vi "MyrioProject.vi"() -> ()   [LabVIEW 2018]
doc: "The myRIO Project template acquires acceleration data from the onboard accelerometer and displays the changes of acceleration values in a waveform chart."
uses:
  <vilib>/myRIO/Common/Instrument Driver Framework/myRIO v1.0/Encoder/typedefs/Encoder Signal Mode.ctl
  <vilib>/Platform/TimedLoop/XDataNode/timing_clust.ctl
  <vilib>/Platform/TimedLoop/XDataNode/nitl_modes.ctl
  <vilib>/Platform/TimedLoop/XDataNode/wakeup.ctl
  <vilib>/Analysis/Matrix/Datatypes/RealMatrix.ctl
  <vilib>/myRIO/Instrument Drivers/Onboard IO/PWM/typedefs/PWM Reference.ctl
  <vilib>/myRIO/Common/Instrument Driver Framework/Utilities/typedefs/myRIO Generic Hardware Reference.ctl
  <vilib>/myRIO/Common/Instrument Driver Framework/Utilities/typedefs/Hardware Version Enum.ctl
  <vilib>/myRIO/Common/Instrument Driver Framework/Utilities/typedefs/myRIO v1.0 Reference.ctl
  <vilib>/myRIO/Common/Instrument Driver Framework/Utilities/typedefs/Generic FPGA Reference.ctl
  <vilib>/myRIO/Common/Instrument Driver Framework/myRIO v1.0/PWM/typedefs/PWM Channels Enum.ctl
  <vilib>/myRIO/Instrument Drivers/Onboard IO/PWM/typedefs/PWM Configuration.ctl
  <vilib>/userdefined/High Color/nirio_resource_hc.ctl
  <vilib>/myRIO/Common/Instrument Driver Framework/myRIO v1.0/Encoder/typedefs/Encoder Configuration v1.0.ctl
  <vilib>/myRIO/Instrument Drivers/Onboard IO/Encoder/typedefs/Encoder Reference.ctl
  <vilib>/myRIO/Common/Instrument Driver Framework/myRIO v1.0/Encoder/typedefs/Encoder Channels Enum.ctl
  <vilib>/myRIO/Instrument Drivers/Onboard IO/DIO/typedefs/DIO Reference.ctl
  <vilib>/myRIO/Common/Instrument Driver Framework/myRIO v1.0/DIO/typedefs/DIO Channels List.ctl
  <vilib>/myRIO/Common/Instrument Driver Framework/myRIO v1.0/DIO/typedefs/DIO Channels Enum.ctl
  <vilib>/myRIO/Instrument Drivers/Onboard IO/AI/typedefs/AI Reference.ctl
  <vilib>/myRIO/Common/Instrument Driver Framework/myRIO v1.0/AI/typedefs/AI Channels List.ctl
  <vilib>/myRIO/Common/Instrument Driver Framework/myRIO v1.0/AI/typedefs/AI Channels Enum.ctl
  <vilib>/myRIO/Common/Instrument Driver Framework/Utilities/typedefs/Analog Scaling Constants List.ctl
  <vilib>/myRIO/Common/Instrument Driver Framework/Utilities/typedefs/Analog Scaling Constants.ctl
  <vilib>/myRIO/Common/Instrument Driver Framework/myRIO v1.0/PWM/vis/myRIO v1.1 Open PWM.vi
  <vilib>/myRIO/Common/Instrument Driver Framework/myRIO v1.0/Encoder/vis/myRIO v1.1 Open Encoder.vi
  <vilib>/myRIO/Common/Instrument Driver Framework/Utilities/vis/Is FPGA Ref Available.vi
  <vilib>/myRIO/Common/Instrument Driver Framework/myRIO v1.0/AI/vis/myRIO v1.1 Open AI.vi
  <vilib>/myRIO/Common/Instrument Driver Framework/myRIO v1.0/DIO/vis/myRIO v1.1 Open DIO.vi
  <vilib>/myRIO/Instrument Drivers/Onboard IO/PWM/vis/Set Duty Cycle and Frequency.vi
  <vilib>/myRIO/Instrument Drivers/Onboard IO/DIO/vis/Write.vi
  <vilib>/myRIO/Common/Instrument Driver Framework/Utilities/vis/Validate Channels.vi
  <vilib>/myRIO/Common/Instrument Driver Framework/myRIO v1.0/PWM/vis/myRIO v1.0 Reserve PWM.vi
  <vilib>/myRIO/Common/Instrument Driver Framework/myRIO v1.0/Encoder/vis/myRIO v1.0 Reserve Encoder.vi
  <vilib>/myRIO/Common/Instrument Driver Framework/myRIO v1.0/AI/vis/myRIO v1.0 Reserve AI.vi
  <vilib>/myRIO/Common/Instrument Driver Framework/myRIO v1.0/DIO/vis/myRIO v1.0 Reserve DIO.vi
  <vilib>/myRIO/Common/Instrument Driver Framework/myRIO v1.0/Encoder/vis/myRIO v1.0 Close Encoder.vi
  <vilib>/myRIO/Common/Instrument Driver Framework/myRIO v1.0/PWM/vis/myRIO v1.0 Close PWM.vi
  <vilib>/myRIO/Common/Instrument Driver Framework/myRIO v1.0/PWM/vis/myRIO v1.0 Build MUX Configuration PWM.vi
  <vilib>/myRIO/Common/Instrument Driver Framework/myRIO v1.0/Resource Manager/vis/myRIO v1.0 Reserve Channel List.vi
  <vilib>/myRIO/Common/Instrument Driver Framework/myRIO v1.0/Encoder/vis/myRIO v1.0 Build MUX Configuration Encoder.vi
  <vilib>/myRIO/Common/Instrument Driver Framework/myRIO v1.0/AI/vis/myRIO v1.0 Build MUX Configuration AI.vi
  <vilib>/myRIO/Common/Instrument Driver Framework/myRIO v1.0/DIO/vis/myRIO v1.0 Build MUX Configuration DIO.vi
  <vilib>/myRIO/Common/Instrument Driver Framework/myRIO v1.0/Encoder/vis/myRIO v1.0 Unreserve Encoder.vi
  <vilib>/myRIO/Common/Instrument Driver Framework/myRIO v1.0/PWM/vis/myRIO v1.0 Unreserve PWM.vi
  <vilib>/myRIO/Common/Instrument Driver Framework/myRIO v1.0/Resource Manager/vis/myRIO v1.0 Create Configuration List.vi
  <vilib>/myRIO/Common/Instrument Driver Framework/myRIO v1.0/Resource Manager/vis/myRIO v1.0 Reserve Channel.vi
  <vilib>/myRIO/Common/Instrument Driver Framework/myRIO v1.0/Resource Manager/vis/myRIO v1.0 Unreserve Channel.vi
  <vilib>/myRIO/Common/Instrument Driver Framework/myRIO v1.0/Resource Manager/vis/myRIO v1.0 Unreserve Channel List.vi
  <vilib>/myRIO/Common/Instrument Driver Framework/myRIO v1.0/Resource Manager/vis/myRIO v1.0 Build Mutex Name.vi
  <vilib>/Utility/VariantDataType/GetNumericInfo.vi
  <vilib>/Utility/error.llb/Error Cluster From Error Code.vi
  <vilib>/myRIO/Common/Instrument Driver Framework/myRIO v1.0/myRIO v1.1 Open.vi
  <vilib>/myRIO/Common/Instrument Driver Framework/Utilities/vis/IO Manager.vi
  <vilib>/myRIO/Common/Instrument Driver Framework/Utilities/vis/Configuration Manager.vi
  <vilib>/myRIO/Common/Instrument Driver Framework/myRIO v1.0/Resource Manager/vis/myRIO v1.0 Configure IO.vi
  <vilib>/myRIO/Common/Instrument Driver Framework/myRIO v1.0/myRIO v1.0 Close.vi
  <vilib>/myRIO/Common/Instrument Driver Framework/myRIO v1.0/PWM/vis/myRIO v1.0 Write PWM.vi
  <vilib>/myRIO/Common/Instrument Driver Framework/myRIO v1.0/Encoder/vis/myRIO v1.0 Configure Encoder.vi
  <vilib>/myRIO/Common/Instrument Driver Framework/myRIO v1.0/Encoder/vis/myRIO v1.0 Enable Encoder.vi
  <vilib>/myRIO/Common/Instrument Driver Framework/myRIO v1.0/DIO/vis/myRIO v1.0 Read DIO.vi
  <vilib>/myRIO/Common/Instrument Driver Framework/myRIO v1.0/AI/vis/myRIO v1.0 Get Scaling Constants AI.vi
  <vilib>/myRIO/Common/Instrument Driver Framework/myRIO v1.0/AI/vis/myRIO v1.0 Read AI.vi
  <vilib>/myRIO/Common/Instrument Driver Framework/myRIO v1.0/Encoder/vis/myRIO v1.0 Read Encoder.vi
  <vilib>/myRIO/Common/Instrument Driver Framework/myRIO v1.0/DIO/vis/myRIO v1.0 Write DIO.vi
  <vilib>/myRIO/Common/Instrument Driver Framework/myRIO v1.0/Encoder/vis/myRIO v1.0 Shutdown Encoder.vi
  <vilib>/myRIO/Common/Instrument Driver Framework/myRIO v1.0/PWM/vis/myRIO v1.0 Shutdown PWM.vi
  <vilib>/platform/TimedLoop/XDataNode/XDataNode.xnode
  <vilib>/myRIO/Instrument Drivers/Onboard IO/PWM/vis/myRIO PWM Open.xnode
  <vilib>/myRIO/Instrument Drivers/Onboard IO/Encoder/vis/myRIO Encoder Open.xnode
  <vilib>/myRIO/Express VI/Onboard Devices/Button/Button Express VI.xnode
  <vilib>/myRIO/Instrument Drivers/Onboard IO/DIO/vis/myRIO DIO Open.xnode
  <vilib>/myRIO/Express VI/Onboard IO/AI/AI Express VI.xnode
  <vilib>/myRIO/Instrument Drivers/Onboard IO/AI/vis/myRIO AI Open.xnode
  <vilib>/myRIO/Express VI/Onboard IO/PWM/PWM Express VI.xnode
  <vilib>/myRIO/Express VI/Onboard IO/DO/DO Express VI.xnode
  <vilib>/myRIO/Instrument Drivers/Onboard IO/Encoder/Encoder.lvlib
  <vilib>/myRIO/Instrument Drivers/Onboard IO/PWM/PWM.lvlib
  <vilib>/myRIO/Instrument Drivers/Onboard IO/DIO/DIO.lvlib
  <vilib>/myRIO/Instrument Drivers/Onboard IO/AI/AI.lvlib
  <vilib>/Platform/TimedLoop/XDataNode/XDNodeRunTimeDep.lvlib
  <vilib>/Analysis/Matrix/NI_Matrix.lvlib
panel:
  out "Waveform Chart 2":cluster{"velocidad":dbl, "Numeric out":dbl}(graph)
  out "Waveform Chart":cluster{"velocidad":dbl, "Numeric out":dbl}(graph)
  in  "pequeoffset":dbl
  in  "s":bool
  in  "grandeoffset":dbl
  in  "saturacion 2":dbl=0.3
  in  "Garra":bool
  out "stall":bool
  in  "Start":bool
  in  "Stop Button":bool
  out "element":dbl
  out "element 2":dbl
  in  "manual":bool
  out "data":dbl
  out "sensor2 (A/AI2 (Pin 7))":dbl
  out "sensor1":dbl
  out "stallRojo (A/AI0 (Pin 3))":dbl
  out "stallBlanco (A/AI1 (Pin 5))":dbl
  out "subarray 2":dbl[][](array[numeric])
  out "subarray":dbl[][](array[numeric])
  out "vectores":dbl[][][](array[numeric])
  in  "saturacion":dbl=0.3
  in  "Garra":dbl(slide)=0.5 scale=0.05..0.1
  in  "Subir":dbl(slide)=0.5 scale=0.05..0.15
  in  "Reset Counter 2":bool
  in  "Reset Counter":bool
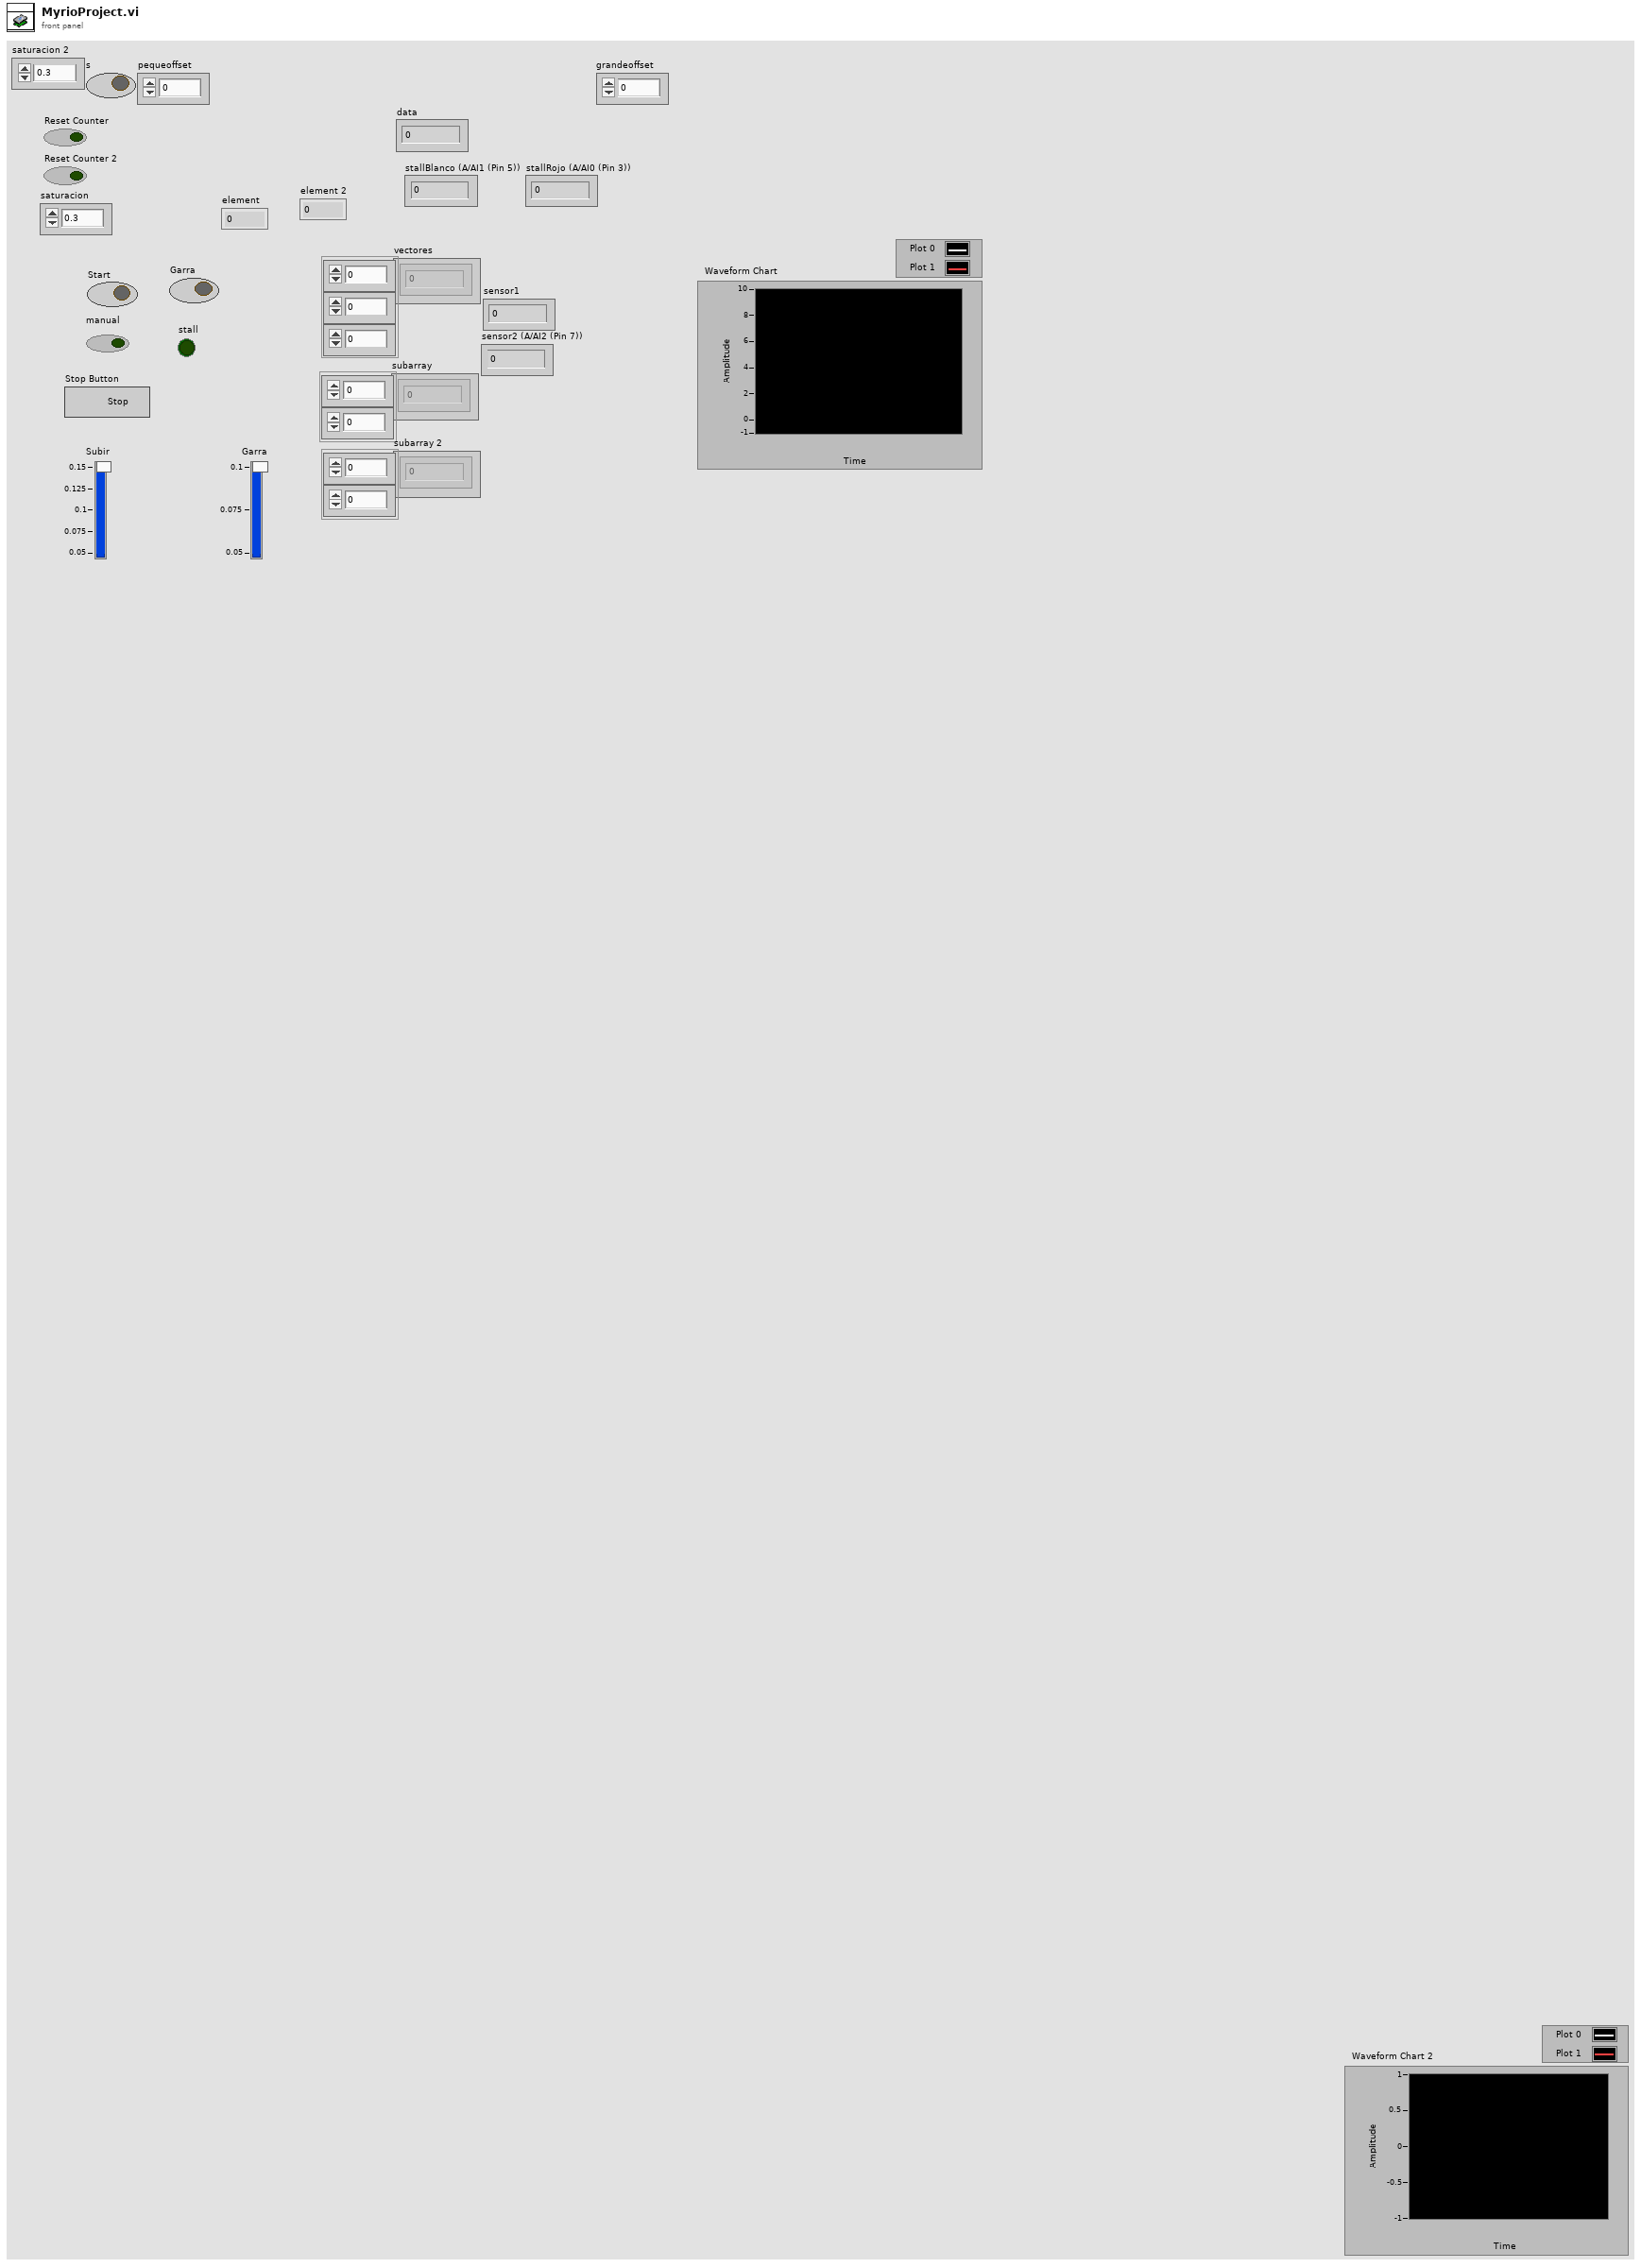
[diagram p1: front panel]
types:
  T1 = typedef "NI_Matrix.lvlib/RealMatrix.ctl" = dbl[][]
  T2 = enum16{"Up-Closed", "Baja-abre", "cierra", "sube"}
  T3 = enum16{"normal", "grande-Sensor", "grande home", "peque-sensor", "peque- home", "peque-reset"}
  T4 = typedef "Encoder Signal Mode.ctl" = enum16{"Quadrature phase signal", "Step and direction signal"}
  T5 = typedef "PWM.lvlib/PWM Reference.ctl" = cluster{"myRIO Reference":T6, "PWM Channels Enum":T10, "PWM Configuration":T11}
  T6 = typedef "myRIO Generic Hardware Reference.ctl" = cluster{"myRIO Model":T7, "myRIO Hardware Reference":T8}
  T7 = typedef "Hardware Version Enum.ctl" = enum16{"Unknown", "myRIO-1900", "myRIO-1950", "roboRIO", "NI ELVIS RIO CM", "ELVIS III"}
  T8 = typedef "myRIO v1.0 Reference.ctl" = cluster{"Generic FPGA Reference":T9, "Allow multiple opens":bool}
  T9 = typedef "Generic FPGA Reference.ctl" = refnum<k20>
  T10 = typedef "PWM Channels Enum.ctl" = enum16{"Not Connected", "C/PWM0", "C/PWM1", "A/PWM0", "A/PWM1", "A/PWM2", "A/PWM3", "A/PWM4", "A/PWM5", "A/PWM6", "A/PWM7", "A/PWM8", "A/PWM9", "A/PWM10", "A/PWM11", "A/PWM12", "A/PWM13", "A/PWM14", "A/PWM15", "A/PWM16", "A/PWM17", "A/PWM18", "A/PWM19", "B/PWM0", "B/PWM1", "B/PWM2", "B/PWM3", "B/PWM4", "B/PWM5", "B/PWM6", "B/PWM7", "B/PWM8", "B/PWM9", "B/PWM10", "B/PWM11", "B/PWM12", "B/PWM13", "B/PWM14", "B/PWM15", "B/PWM16", "B/PWM17", "B/PWM18", "B/PWM19", "PWM/PWM0", "PWM/PWM1", "PWM/PWM2", "PWM/PWM3", "PWM/PWM4", "PWM/PWM5", "PWM/PWM6", "PWM/PWM7", "PWM/PWM8", "PWM/PWM9"}
  T11 = typedef "PWM.lvlib/PWM Configuration.ctl" = cluster{"Frequency":dbl, "Duty Cycle":dbl}
  T12 = typedef "Encoder.lvlib/Encoder Reference.ctl" = cluster{"myRIO Reference":T6, "Encoder Channels Enum":T13}
  T13 = typedef "Encoder Channels Enum.ctl" = enum16{"Not Connected", "C/ENC0", "C/ENC1", "A/ENC", "A/ENC0", "A/ENC1", "A/ENC2", "A/ENC3", "A/ENC4", "A/ENC5", "A/ENC6", "A/ENC7", "A/ENC8", "A/ENC9", "B/ENC", "B/ENC0", "B/ENC1", "B/ENC2", "B/ENC3", "B/ENC4", "B/ENC5", "B/ENC6", "B/ENC7", "B/ENC8", "B/ENC9", "DIO/ENC0", "DIO/ENC1", "DIO/ENC2", "DIO/ENC3", "DIO/ENC4"}
  T14 = cluster{"Double":dbl, "dbl Scaled Value":dbl, "Output":dbl, "seconds since 1Jan1904":timestamp, dbl, dbl, dbl}
  T15 = typedef "XDNodeRunTimeDep.lvlib/timing_clust.ctl" = cluster{"Expected End [f-1]":u64, "Actual End [f-1]":u64, "Finished Late? [f-1]":bool, "Expected End [i-1]":u64, "Actual End [i-1]":u64, "Finished Late? [i-1]":bool, "Expected Start [i]":u64, "Actual Start [i]":u64, "Expected Start [f]":u64, "Actual Start [f]":u64, "Source Name":string, "Structure Name":string, "Period":i64, "Deadline":i64, "Offset":i64, "Start":i64, "Priority":i32, "Timeout":i32, "Mode":T16, "Wakeup Reason":T17, "Error":errorcluster, "Source Type":string, "Secondary Source Type":string, "Global End Time":u64, "Global Start Time":u64, "Frame Duration":u64, "Iteration Duration":u64, "Assigned CPU":i32, "I/O Scan Engine Mode":u32}
  T16 = typedef "XDNodeRunTimeDep.lvlib/nitl_modes.ctl" = enum32{"No Change", "Process missed periods, maintain original phase", "Discard missed periods, maintain original phase", "Process missed periods, ignore original phase", "Discard missed periods, ignore original phase"}
  T17 = typedef "XDNodeRunTimeDep.lvlib/wakeup.ctl" = enum32{"Normal", "Aborted", "Asynchronous wakeup", "Timing source error", "Timed loop error", "Timeout"}
  T18 = typedef "nirio_resource_hc.ctl" = tag
  T19 = typedef "AI.lvlib/AI Reference.ctl" = cluster{"myRIO Reference":T6, "AI Channels List":T20, "AI Scaling Constants List":T22}
  T20 = typedef "AI Channels List.ctl" = T21[]
  T21 = typedef "AI Channels Enum.ctl" = enum16{"Not Connected", "AudioIn/Left", "AudioIn/Right", "C/AI0", "C/AI1", "A/AI0", "A/AI1", "A/AI2", "A/AI3", "A/AI4", "A/AI5", "A/AI6", "A/AI7", "B/AI0", "B/AI1", "B/AI2", "B/AI3", "B/AI4", "B/AI5", "B/AI6", "B/AI7", "AI/AI0", "AI/AI1", "AI/AI2", "AI/AI3", "A/AI0 (DIFF)", "A/AI1 (DIFF)", "A/AI2 (DIFF)", "A/AI3 (DIFF)", "B/AI0 (DIFF)", "B/AI1 (DIFF)", "B/AI2 (DIFF)", "B/AI3 (DIFF)"}
  T22 = typedef "Analog Scaling Constants List.ctl" = T23[]
  T23 = typedef "Analog Scaling Constants.ctl" = cluster{"LSB Weight (Volts)":dbl, "Offset (Volts)":dbl, "Signed?":bool}
  T24 = typedef "DIO.lvlib/DIO Reference.ctl" = cluster{"myRIO Reference":T6, "DIO Channels List":T25}
  T25 = typedef "DIO Channels List.ctl" = T26[]
  T26 = typedef "DIO Channels Enum.ctl" = enum16{"Not Connected", "C/DIO0", "C/DIO1", "C/DIO2", "C/DIO3", "C/DIO4", "C/DIO5", "C/DIO6", "C/DIO7", "A/DIO0", "A/DIO1", "A/DIO2", "A/DIO3", "A/DIO4", "A/DIO5", "A/DIO6", "A/DIO7", "A/DIO8", "A/DIO9", "A/DIO10", "A/DIO11", "A/DIO12", "A/DIO13", "A/DIO14", "A/DIO15", "A/DIO16", "A/DIO17", "A/DIO18", "A/DIO19", "B/DIO0", "B/DIO1", "B/DIO2", "B/DIO3", "B/DIO4", "B/DIO5", "B/DIO6", "B/DIO7", "B/DIO8", "B/DIO9", "B/DIO10", "B/DIO11", "B/DIO12", "B/DIO13", "B/DIO14", "B/DIO15", "B/DIO16", "B/DIO17", "B/DIO18", "B/DIO19", "LED0", "LED1", "LED2", "LED3", "Button0", "DIO/DIO0", "DIO/DIO1", "DIO/DIO2", "DIO/DIO3", "DIO/DIO4", "DIO/DIO5", "DIO/DIO6", "DIO/DIO7", "DIO/DIO8", "DIO/DIO9", "SPI/CS0", "SPI/CS1", "SPI/CS2", "SPI/CS3", "LED RADIO (Green)", "LED RADIO (Red)", "LED COMM (Green)", "LED COMM (Red)", "LED MODE (Green)", "LED MODE (Red)"}
  T27 = cluster{dbl, "saturacion":dbl, dbl, "seconds since 1Jan1904":timestamp, dbl, "saturacion 2":dbl, dbl}
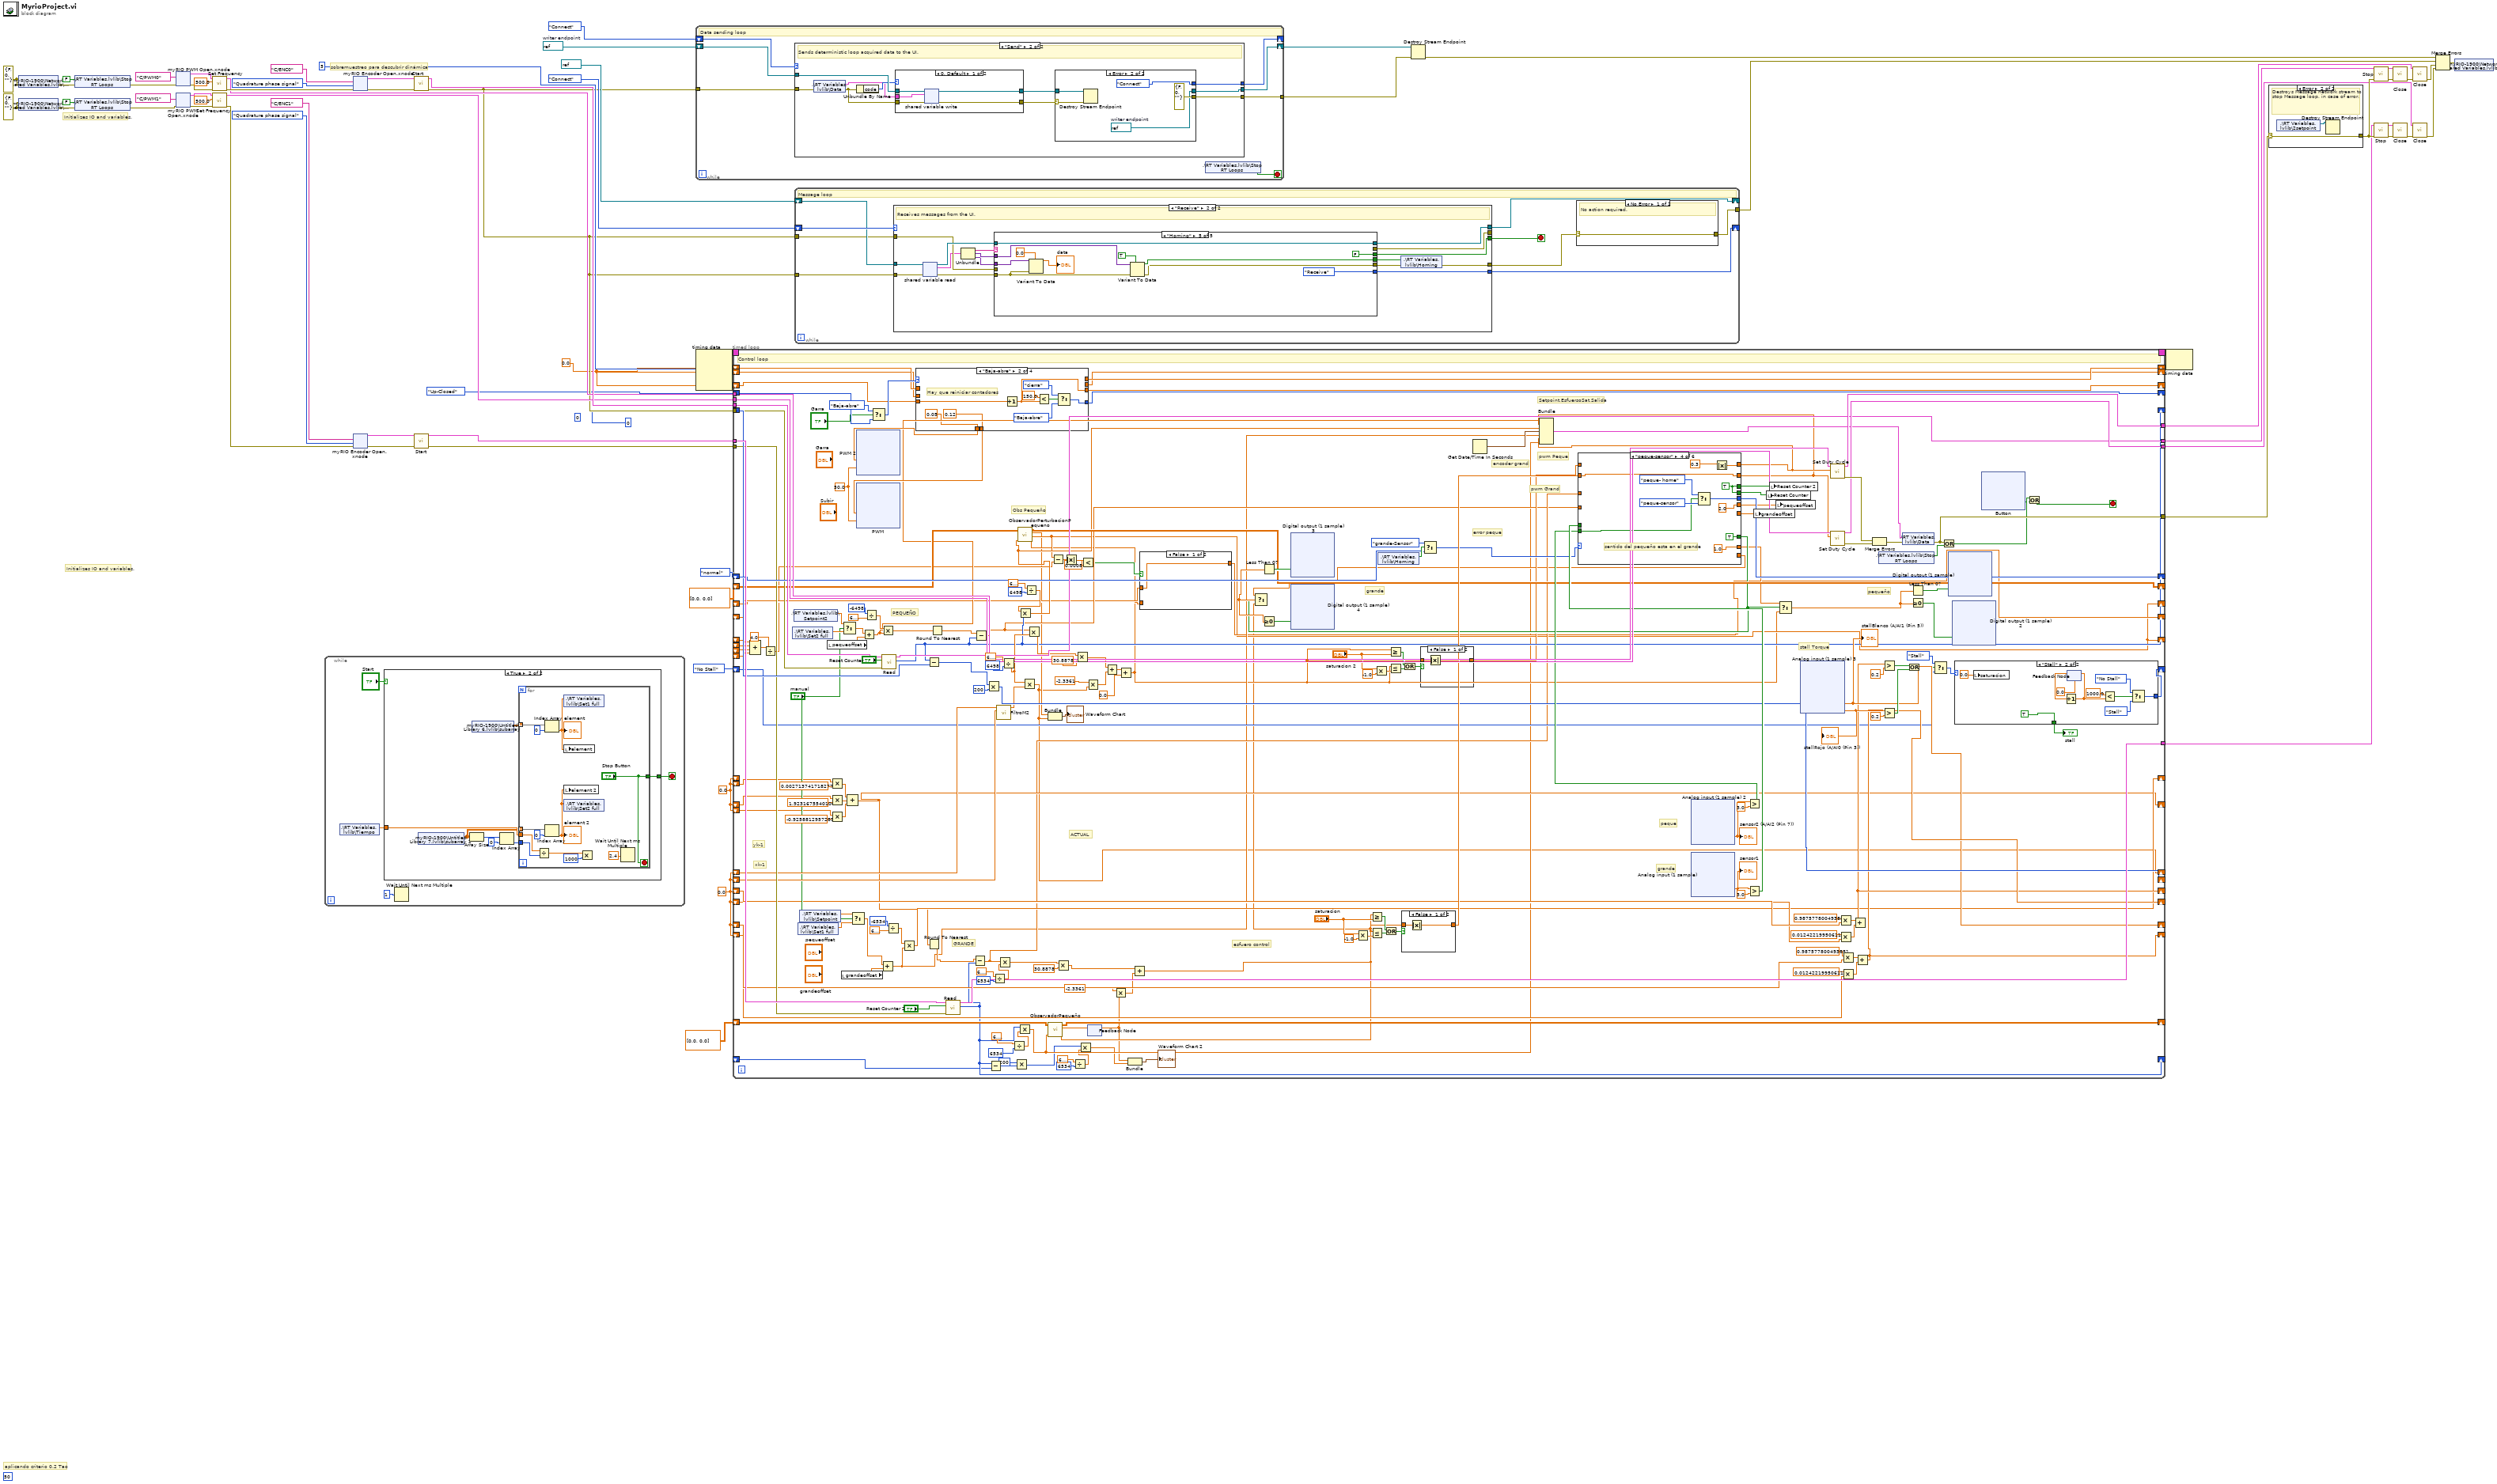
[diagram p0: block diagram]
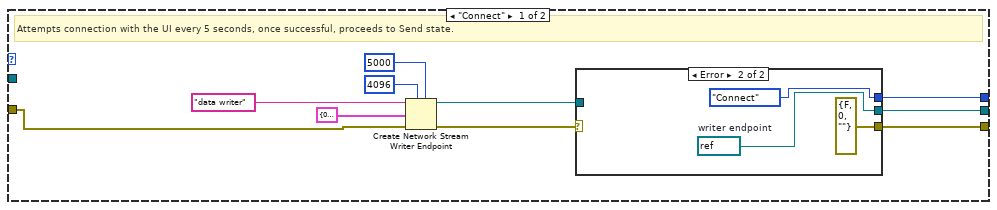
[diagram p4: hidden frame]
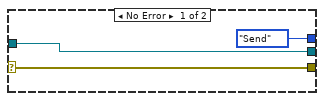
[diagram p5: hidden frame]
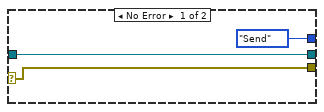
[diagram p6: hidden frame]
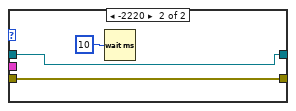
[diagram p7: hidden frame]
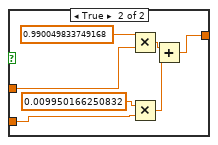
[diagram p8: hidden frame]
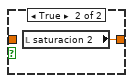
[diagram p9: hidden frame]
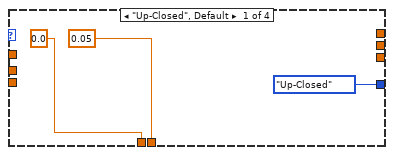
[diagram p10: hidden frame]
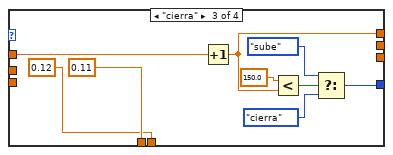
[diagram p11: hidden frame]
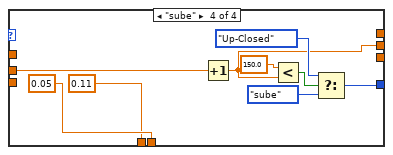
[diagram p12: hidden frame]
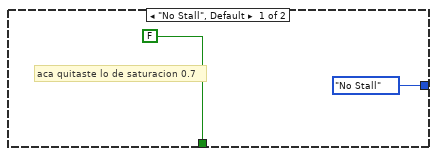
[diagram p13: hidden frame]
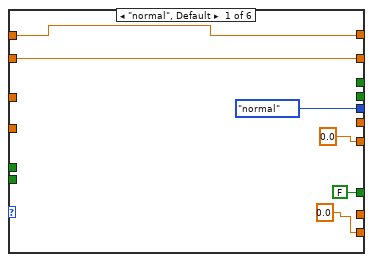
[diagram p14: hidden frame]
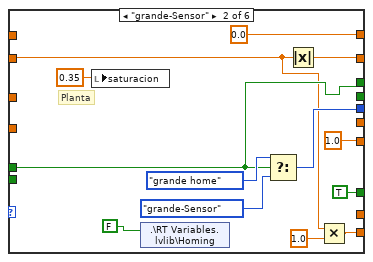
[diagram p15: hidden frame]
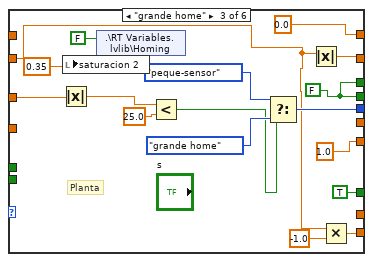
[diagram p16: hidden frame]
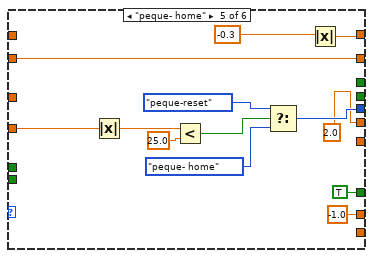
[diagram p17: hidden frame]
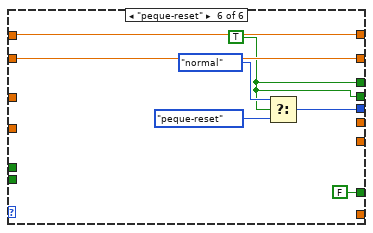
[diagram p18: hidden frame]
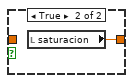
[diagram p19: hidden frame]
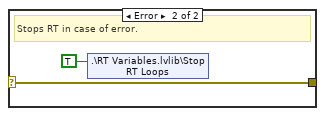
[diagram p20: hidden frame]
diagram:
  w2 = 0.0
  w3 = 0.0
  w6 = 0.0
  (unwired) 0
  (unwired) 50
  w21 = refnum<k21> refnum  # writer endpoint
  w34 = errorcluster {"status"=FALSE, "code"=0, "source"=""} ("error IO")
  w56 = errorcluster {"status"=FALSE, "code"=0, "source"=""} ("error IO")
  # "aplicando criterio 0.2 Tao"
  # "sobremuestreo para descubrir dinámica"
  # "Initializes IO and variables."
  # "Initializes IO and variables."
  n1 = shared-variable "myRIO-1900\\Network Shared Variables.lvlib\\error IO"(w56, error in=w56) -> (error out=w57:errorcluster)
  n2 = shared-variable "myRIO-1900\\Network Shared Variables.lvlib\\error IO"(w34, error in=w34) -> (error out=w35:errorcluster)
  n3 = shared-variable ".\\RT Variables.lvlib\\Stop RT Loops"(FALSE ("Stop RT Loops"), error in=w57) -> (error out=w44:errorcluster)
  n4 = shared-variable ".\\RT Variables.lvlib\\Stop RT Loops"(FALSE ("Stop RT Loops"), error in=w35) -> (error out=w27:errorcluster)
  n5 = xnode "myRIO PWM Open.xnode"("error in (no error)"=w44, "Channel Name"=tag "C/PWM0") -> ("error out"=w46:errorcluster, "PWM Ref Out"=w45:T5)  [unwired: 1 in]
  n6 = xnode "myRIO PWM Open.xnode"("error in (no error)"=w27, "Channel Name"=tag "C/PWM1") -> ("error out"=w29:errorcluster, "PWM Ref Out"=w28:T5)  [unwired: 1 in]
  n7 = call <vilib>:"Set Frequency.vi"("error in (no error)"=w46, "Frequency [Hz]"=500.0, "PWM Ref In"=w45) -> ("error out"=w43:errorcluster, "PWM Ref Out"=w40:T5)  [unwired: 6 in]
  n8 = call <vilib>:"Set Frequency.vi"("error in (no error)"=w29, "Frequency [Hz]"=500.0, "PWM Ref In"=w28) -> ("error out"=w26:errorcluster, "PWM Ref Out"=w22:T5)  [unwired: 6 in]
  n9 = while {
    stop <- w68 stop-if-true
    n10 = shared-variable ".\\RT Variables.lvlib\\Tiempo"() -> (w70:dbl)  [unwired: 1 in, 1 out]
    n11 = case shown="True" "Start" {
      tunnel: w70 -> [_ w77]
      tunnel: [_ w76] -> w68
      frame False {
      }
      frame True {
        n12 = shared-variable "myRIO-1900\\Untitled Library 7.lvlib\\subarray 2"() -> (w75:dbl[][])  [unwired: 1 in, 1 out]
        n13 = Array Size(array=w75) -> (size(s)=w73:i32[])
        n14 = shared-variable "myRIO-1900\\Untitled Library 6.lvlib\\subarray"() -> (w78:dbl[][])  [unwired: 1 in, 1 out]
        n15 = Index Array(array=w73, index=0) -> (element=w72:i32)
        n16 = for {
          tunnel: w78 -> [w88] mode=indexing
          tunnel: w75 -> [w85] mode=indexing
          tunnel: w77 -> [w82]
          tunnel: ["Stop Button"] -> w76
          tunnel: w72 -> [w80]
          stop <- "Stop Button" stop-if-true
          n17 = Divide(x=w82, y=w80) -> (x/y=w90:dbl)
          n18 = Index Array(array=w88, index=0) -> (element=w84:dbl)
          "element" <- w84
          n19 = Index Array(array=w85, index=0) -> (element=w83:dbl)
          "element 2" <- w83
          n20 = shared-variable ".\\RT Variables.lvlib\\Set1 full"(w84) -> ()  [unwired: 1 in, 1 out]
          n21 = local write "element"(w84) -> ()
          n22 = local write "element 2"(w83) -> ()
          n23 = shared-variable ".\\RT Variables.lvlib\\Set2 full"(w83) -> ()  [unwired: 1 in, 1 out]
          n24 = Multiply(x=w90, y=1000) -> ()  [unwired: 1 out]
          n25 = Wait Until Next ms Multiple(millisecond multiple=2.4) -> ()  [unwired: 1 out]
        }
      }
    }
    n26 = Wait Until Next ms Multiple(millisecond multiple=u32 1) -> ()  [unwired: 1 out]
  }
  n27 = xnode "myRIO Encoder Open.xnode"("error in (no error)"=w43, "Channel Name"=tag "C/ENC0", "Encoder Signal Mode"=Encoder_Signal_Mode."Quadrature phase signal") -> ("error out"=w53:errorcluster, "Encoder Ref Out"=w52:T12)  [unwired: 2 in]
  n28 = xnode "myRIO Encoder Open.xnode"("error in (no error)"=w26, "Channel Name"=tag "C/ENC1", "Encoder Signal Mode"=Encoder_Signal_Mode."Quadrature phase signal") -> ("error out"=w32:errorcluster, "Encoder Ref Out"=w31:T12)  [unwired: 2 in]
  n29 = call <vilib>:"Start.vi"("error in (no error)"=w53, "Encoder Ref In"=w52) -> ("error out"=w11:errorcluster, "Encoder Ref Out"=w50:T12)  [unwired: 8 in]
  n30 = call <vilib>:"Start.vi"("error in (no error)"=w32, "Encoder Ref In"=w31) -> ("error out"=w10:errorcluster, "Encoder Ref Out"=w23:T12)  [unwired: 8 in]
  n31 = while {
    shift-right: [w95] -> w62
    shift-left: w21 -> [w93]
    tunnel: [w94] -> w63
    tunnel: w11 -> [w92]
    shift-right: [w91] -> _
    shift-left: enum16{"Connect", "Send"}."Connect" ("Message states") -> [w96]
    stop <- w97 stop-if-true
    # "Data sending loop"
    n32 = case shown="\"Send\"" w96 {
      tunnel: [w101 w116] -> w94
      tunnel: [w99 w114] -> w95
      tunnel: [w105 w117] -> w91
      tunnel: w93 -> [_ w123]
      tunnel: w92 -> [w102 w122]
      frame "Connect" {
        # "Attempts connection with the UI every 5 seconds, once successful, proceeds to Send state."
        n33 = Create Network Stream Writer Endpoint(5:5000 ("timeout in ms (-1)"), 7:4096 ("writer buffer size"), 8:w102, 9:T14 {"Double"=0.0, "dbl Scaled Value"=0.0, "Output"=0.0, "seconds since 1Jan1904"=timestamp(0 s since 1904-01-01), 0.0, 0.0, 0.0} ("Data"), 11:"data writer" ("writer name")) -> (0:w103:errorcluster, 3:w100:refnum<k21>)  [unwired: 2 in]
        n34 = case shown="Error" w103 {
          selector: w103 -> [w108 _]
          tunnel: [enum16{"Connect", "Send"}."Send" ("Message states") enum16{"Connect", "Send"}."Connect" ("Message states")] -> w105
          tunnel: [w108 errorcluster {"status"=FALSE, "code"=0, "source"=""} ("error IO")] -> w101
          tunnel: w100 -> [w110 _]
          tunnel: [w110 w111] -> w99
          frame No Error {
          }
          frame Error {
            w111 = refnum<k21> refnum  # writer endpoint
          }
        }
      }
      frame "Send" {
        # "Sends deterministic loop acquired data to the UI."
        n35 = shared-variable ".\\RT Variables.lvlib\\Data"(error in=w122) -> (w119:T14, error out=w121:errorcluster)
        n36 = Unbundle By Name(w121) -> ("code"=w120:i32)
        n37 = case shown="0, Default" w120 {
          tunnel: [w136 w138] -> w118
          tunnel: [w135 w137] -> w115
          tunnel: w123 -> [w134 w137]
          tunnel: w121 -> [w133 w138]
          tunnel: w119 -> [w132 _]
          frame 0, Default {
            n38 = shared-variable-write(w134, w133, w132) -> (w135:refnum<k21>, w136:errorcluster)  [unwired: 1 in, 1 out]
          }
          frame -2220 {
            n39 = Wait (ms)(milliseconds to wait=u32 10) -> ()  [unwired: 1 out]
          }
        }
        n40 = case shown="Error" w118 {
          selector: w118 -> [w126 w130]
          tunnel: [enum16{"Connect", "Send"}."Send" ("Message states") enum16{"Connect", "Send"}."Connect" ("Message states")] -> w117
          tunnel: [w126 errorcluster {"status"=FALSE, "code"=0, "source"=""} ("error IO")] -> w116
          tunnel: w115 -> [w124 w129]
          tunnel: [w124 w127] -> w114
          frame No Error {
          }
          frame Error {
            w127 = refnum<k21> refnum  # writer endpoint
            n41 = Destroy Stream Endpoint(8:w130, 11:w129) -> ()  [unwired: 1 out]
          }
        }
      }
    }
    n42 = shared-variable ".\\RT Variables.lvlib\\Stop RT Loops"() -> (w97:bool)  [unwired: 1 in, 1 out]
  }
  n43 = node-c288(i64 5 ("Period")) -> (w67:T15)  [unwired: 3 in]
  n44 = timed-loop {
    timing: w67 -> [_]
    timing-out: [_] -> w66
    tunnel: [w342] -> w55
    tunnel: w50 -> [w324]
    tunnel: [w323] -> w47
    tunnel: w40 -> [w314]
    tunnel: [w341] -> w39
    tunnel: w23 -> [w338]
    tunnel: w22 -> [w337]
    tunnel: [w333] -> w16
    tunnel: [w332] -> w15
    shift-right: [w313] -> _
    shift-left: T3."normal" ("Enum") -> [w312]
    shift-right: [w209] -> _
    shift-left: 0 -> [w302]
    tunnel: w10 -> [w300]
    tunnel: w11 -> [w299]
    shift-right: [w275] -> _
    shift-left: w6 -> [w274]
    shift-right: [w140] -> _
    shift-left: w6 -> [w273]
    shift-right: [w269] -> _
    shift-left: T1 [[0.0], [0.0]] ("A + B") -> [w268]
    shift-right: [w248] -> _
    shift-left: w6 -> [w258]
    shift-right: [w247] -> _
    shift-left: w6 -> [w253]
    shift-right: [w252] -> _
    shift-left: w6 -> [w251]
    shift-right: [w250] -> _
    shift-left: w6 -> [w249]
    shift-right: [w239] -> _
    shift-left: enum16{"No Stall", "Stall"}."No Stall" -> [w238]
    shift-right: [w234] -> _
    shift-left: T2."Up-Closed" -> [w233]
    shift-right: [w230] -> _
    shift-left: w3 -> [w231]
    shift-right: [w226] -> _
    shift-left: w3 -> [w229]
    shift-right: [w227] -> _
    shift-left: w3 -> [w228]
    shift-right: [w212] -> _
    shift-left: w2 -> [_]
    shift-right: [w210] -> _
    shift-left: w2 -> [w216]
    shift-left: w2 -> [w217]
    shift-left: w2 -> [w215]
    shift-right: [w172] -> _
    shift-left: _ -> [w183]
    shift-left: _ -> [w182]
    shift-left: _ -> [w181]
    shift-left: _ -> [w168]
    shift-right: [w174] -> _
    shift-left: _ -> [w173]
    shift-right: [w172] -> _
    shift-left: _ -> [w171]
    shift-right: [w160] -> _
    shift-left: T1 [[0.0], [0.0]] ("A + B") -> [w161]
    shift-right: [w154] -> _
    shift-left: _ -> [w153]
    stop <- w330 stop-if-true
    w301 = 50.0 ("Frequency [Hz]")
    # "grande"
    # "pequeño"
    # "ACTUAL"
    # "error peque"
    # "encoder grand"
    # "pwm Grand"
    # "pwm Peque"
    # "esfuero control"
    # "Obs Pequeño"
    # "yk-1"
    # "xk-1"
    # "PEQUEÑO"
    # "peque"
    # "grande"
    # "stall Torque"
    # "Setpoint,EsfuersoSat,Salida"
    # "GRANDE"
    # "Control loop"
    n45 = Compound Arithmetic op=ADD(w183, w182, w181, w168) -> (w180:dbl)
    n46 = Divide(x=w180, y=4.0) -> (x/y=w167:dbl)
    n47 = shared-variable ".\\RT Variables.lvlib\\Set2 full"() -> (w266:dbl)  [unwired: 1 in, 1 out]
    n48 = shared-variable ".\\RT Variables.lvlib\\Setpoint2"() -> (w267:dbl)  [unwired: 1 in, 1 out]
    n49 = shared-variable ".\\RT Variables.lvlib\\Set1 full"() -> (w264:dbl)  [unwired: 1 in, 1 out]
    n50 = shared-variable ".\\RT Variables.lvlib\\Setpoint"() -> (w265:dbl)  [unwired: 1 in, 1 out]
    n51 = local read "pequeoffset"() -> (w194:dbl)
    n52 = Multiply(x=w217, y=0.002713741718277) -> (x*y=w219:dbl)
    n53 = Multiply(x=w216, y=1.923167554010684) -> (x*y=w220:dbl)
    n54 = Multiply(x=w215, y=-0.925881295728961) -> (x*y=w218:dbl)
    n55 = local read "grandeoffset"() -> (w198:dbl)
    n56 = Select(t=w267, s="manual", f=w266) -> (s? t:f=w195:dbl)
    n57 = Compound Arithmetic op=ADD(w219, w220, w218) -> (w210:dbl)
    n58 = Select(t=w265, s="manual", f=w264) -> (s? t:f=w199:dbl)
    n59 = Add(x=w195, y=w194) -> (x+y=w188:dbl)
    n60 = Divide(x=-6498, y=6.283185307179586) -> (x/y=w294:dbl)
    n61 = Select(t=T2."Baja-abre", s="Garra", f=w233) -> (s? t:f=w236:T2)
    n62 = Add(x=w199, y=w198) -> (x+y=w187:dbl)
    n63 = Multiply(x=w294, y=w188) -> (x*y=w189:dbl)
    n64 = call <vilib>:"Read.vi"("error in (no error)"=w299, "Reset Counter"="Reset Counter", "Encoder Ref In"=w324) -> ("Counter Value"=w209:i32, "Encoder Ref Out"=w323:T12)  [unwired: 4 in, 3 out]
    n65 = Divide(x=-6534, y=6.283185307179586) -> (x/y=w291:dbl)
    n66 = Multiply(x=w291, y=w187) -> (x*y=w212:dbl)
    n67 = case shown="\"Baja-abre\"" w236 {
      tunnel: [T2."Up-Closed" w365 w374 w383] -> w234
      tunnel: [0.0 0.05 0.11 0.11] -> w225
      tunnel: [0.05 0.12 0.12 0.05] -> w224
      tunnel: w231 -> [_ _ w369 _]
      tunnel: [_ _ w368 _] -> w230
      tunnel: w229 -> [_ _ _ w379]
      tunnel: w228 -> [_ w361 _ _]
      tunnel: [_ w360 _ _] -> w227
      tunnel: [_ _ _ w378] -> w226
      frame "Up-Closed", Default {
      }
      frame "Baja-abre" {
        # "Hay que reiniciar contadores"
        n68 = Increment(x=w361) -> (x+1=w360:dbl)
        n69 = Less?(x=150.0, y=w360) -> (x < y?=w362:bool)
        n70 = Select(t=T2."cierra", s=w362, f=T2."Baja-abre") -> (s? t:f=w365:T2)
      }
      frame "cierra" {
        n71 = Increment(x=w369) -> (x+1=w368:dbl)
        n72 = Less?(x=150.0, y=w368) -> (x < y?=w372:bool)
        n73 = Select(t=T2."sube", s=w372, f=T2."cierra") -> (s? t:f=w374:T2)
      }
      frame "sube" {
        n74 = Increment(x=w379) -> (x+1=w378:dbl)
        n75 = Less?(x=150.0, y=w378) -> (x < y?=w380:bool)
        n76 = Select(t=T2."Up-Closed", s=w380, f=T2."sube") -> (s? t:f=w383:T2)
      }
    }
    n77 = xnode "PWM 2"("Duty Cycle"=w225, "Frequency [Hz]"=w301) -> ()  [unwired: 1 in, 1 out]
    n78 = xnode "PWM"("Duty Cycle"=w224, "Frequency [Hz]"=w301) -> ()  [unwired: 1 in, 1 out]
    n79 = Subtract(x=w209, y=w302) -> (x-y=w284:i32)
    n80 = Round To Nearest(number=w210) -> (nearest integer value=w327:dbl)
    n81 = Round To Nearest(number=w189) -> (nearest integer value=w322:dbl)
    n82 = call <vilib>:"Read.vi"("error in (no error)"=w300, "Reset Counter"="Reset Counter 2", "Encoder Ref In"=w338) -> ("Counter Value"=w154:i32, "Encoder Ref Out"=w333:T12)  [unwired: 4 in, 3 out]
    n83 = Subtract(x=w327, y=w154) -> (x-y=w201:dbl)
    n84 = Subtract(x=w322, y=w209) -> (x-y=w200:dbl)
    n85 = Multiply(x=w284, y=200) -> (x*y=w275:i32)
    n86 = Subtract(x=w154, y=w153) -> (x-y=w152:i32)
    n87 = Divide(x=6.283185307179586, y=6534) -> (x/y=w276:dbl)
    n88 = call "FiltroM2.vi"("Numeric 3"=w274, "Numeric in"=w273) -> ("Numeric out"=w149:dbl)  [unwired: 9 in]
    n89 = Multiply(x=w201, y=w276) -> (x*y=w165:dbl)
    n90 = Divide(x=6.283185307179586, y=6498) -> (x/y=w278:dbl)
    n91 = Divide(x=6.283185307179586, y=6534) -> (x/y=w186:dbl)
    n92 = Multiply(x=200, y=w152) -> (x*y=w145:i32)
    n93 = Multiply(x=w154, y=w186) -> (x*y=w159:dbl)
    n94 = Multiply(x=w278, y=w149) -> (x*y=w140:dbl)
    n95 = Divide(x=6.283185307179586, y=6498) -> (x/y=w270:dbl)
    n96 = Multiply(x=w270, y=w209) -> (x*y=w211:dbl)
    n97 = Multiply(x=w200, y=w278) -> (x*y=w244:dbl)
    n98 = Multiply(x=w165, y=30.8878) -> (x*y=w162:dbl)
    n99 = Divide(x=6.283185307179586, y=6534) -> (x/y=w146:dbl)
    n100 = Multiply(x=w244, y=30.8878) -> (x*y=w303:dbl)
    n101 = Multiply(x=w145, y=w146) -> (x*y=w144:dbl)
    n102 = Multiply(x=-2.3361, y=w140) -> (x*y=w277:dbl)
    n103 = feedback #1() -> (w141:dbl)  [unwired: 1 in]
    n104 = Add(x=w303, y=w277) -> (x+y=w170:dbl)
    n105 = Multiply(x=-2.3361, y=w141) -> (x*y=w163:dbl)
    n106 = Add(x=w170, y=0.0) -> (x+y=w169:dbl)
    n107 = call "ObservadorPerturbacionPequeno.vi"("entrada planta"=w169, "salida planta"=w211, "xk +1"=w268) -> ("Perturbacion"=w172:dbl, "velocidad"=w155:dbl, "xk"=w269:T1)  [unwired: 6 in]
    n108 = Bundle("velocidad"=w155, w140) -> (→"Waveform Chart":cluster{"velocidad":dbl, dbl})  [unwired: 1 in]
    n109 = Subtract(x=w172, y=w167) -> (x-y=w178:dbl)
    n110 = Absolute Value(x=w178) -> (abs(x)=w177:dbl)
    n111 = Less?(x=w177, y=0.0008) -> (x < y?=w175:bool)
    n112 = Bundle("velocidad"=w141, w144) -> (→"Waveform Chart 2":cluster{"velocidad":dbl, dbl})  [unwired: 1 in]
    n113 = Add(x=w162, y=w163) -> (x+y=w158:dbl)
    n114 = call "ObservadorPequeño.vi"("entrada planta"=w158, "salida planta"=w159, "xk +1"=w161) -> ("velocidad"=w142:dbl, "xk"=w160:T1)  [unwired: 6 in, 1 out]
    n115 = feedback-in #1(w142) -> ()
    n116 = case shown="False" w175 {
      tunnel: [w345 w349] -> w174
      tunnel: w171 -> [_ w348]
      tunnel: w173 -> [w345 w347]
      frame False {
      }
      frame True {
        n117 = Multiply(x=0.990049833749168, y=w347) -> (x*y=w350:dbl)
        n118 = Multiply(x=0.009950166250832, y=w348) -> (x*y=w351:dbl)
        n119 = Add(x=w350, y=w351) -> (x+y=w349:dbl)
      }
    }
    n120 = Multiply(x="saturacion", y=-1.0) -> (x*y=w288:dbl)
    n121 = Greater Or Equal?(x=w158, y="saturacion") -> (x >= y?=w329:bool)
    n122 = Less Or Equal?(x=w158, y=w288) -> (x <= y?=w328:bool)
    n123 = Multiply(x="saturacion 2", y=-1.0) -> (x*y=w205:dbl)
    n124 = shared-variable ".\\RT Variables.lvlib\\Homing"() -> (w315:bool)  [unwired: 1 in, 1 out]
    n125 = Or(x=w329, y=w328) -> (x .or. y?=w157:bool)
    n126 = Greater Or Equal?(x=w169, y="saturacion 2") -> (x >= y?=w203:bool)
    n127 = Less Or Equal?(x=w169, y=w205) -> (x <= y?=w204:bool)
    n128 = case shown="False" w157 {
      tunnel: [w787 w789] -> w310
      tunnel: w158 -> [w788 _]
      frame False {
        n129 = Absolute Value(x=w788) -> (abs(x)=w787:dbl)
      }
      frame True {
        n130 = local read "saturacion"() -> (w789:dbl)
      }
    }
    n131 = Or(x=w203, y=w204) -> (x .or. y?=w208:bool)
    n132 = case shown="False" w208 {
      tunnel: [w353 w355] -> w202
      tunnel: w169 -> [w354 _]
      frame False {
        n133 = Absolute Value(x=w354) -> (abs(x)=w353:dbl)
      }
      frame True {
        n134 = local read "saturacion 2"() -> (w355:dbl)
      }
    }
    n135 = Select(t=T3."grande-Sensor" ("Enum"), s=w315, f=w312) -> (s? t:f=w280:T3)
    n136 = Get Date/Time In Seconds() -> (seconds since 1Jan1904=w344:timestamp)
    n137 = xnode "Analog input (1 sample) 2"() -> ("sensor2 (A/AI2 (Pin 7))"=w297:dbl)  [unwired: 1 in, 1 out]
    "sensor2 (A/AI2 (Pin 7))" <- w297
    n138 = xnode "Analog input (1 sample)"() -> ("A/AI3 (Pin 9)"=w298:dbl)  [unwired: 1 in, 1 out]
    "sensor1" <- w298
    n139 = Greater?(x=w297, y=3.0) -> (0:w309:bool)
    n140 = Greater?(x=w298, y=3.0) -> (0:w311:bool)
    n141 = case shown="\"peque-sensor\"" w280 {
      tunnel: w202 -> [w471 _ _ _ _ w531]
      tunnel: [T3."normal" ("Enum") w486 w503 w514 w527 w533] -> w313
      tunnel: w311 -> [_ w481 _ _ _ _]
      tunnel: w310 -> [w473 w475 w488 w504 w515 w530]
      tunnel: [w473 w479 w493 w504 w515 w530] -> w190
      tunnel: w309 -> [_ _ _ w510 _ _]
      tunnel: [w471 0.0 ("f") 0.0 w508 w520 w531] -> w191
      tunnel: [_ _ w496 w511 _ w529] -> w307
      tunnel: [_ w481 w496 w511 _ w529] -> w305
      tunnel: [FALSE TRUE TRUE TRUE TRUE FALSE] -> w245
      tunnel: w201 -> [_ _ w495 _ _ _]
      tunnel: [0.0 w476 w489 _ _ _] -> w193
      tunnel: w200 -> [_ _ _ _ w519 _]
      tunnel: [0.0 1.0 1.0 _ _ _] -> w197
      tunnel: [_ _ _ 2.0 2.0 _] -> w196
      tunnel: [_ _ _ 1.0 -1.0 _] -> w192
      frame "normal", Default {
      }
      frame "grande-Sensor" {
        # "Planta"
        n142 = local write "saturacion"(0.35 ("f")) -> ()
        n143 = shared-variable ".\\RT Variables.lvlib\\Homing"(FALSE) -> ()  [unwired: 1 in, 1 out]
        n144 = Select(t=T3."grande home" ("Enum"), s=w481, f=T3."grande-Sensor" ("Enum")) -> (s? t:f=w486:T3)
        n145 = Absolute Value(x=w475) -> (abs(x)=w479:dbl)
        n146 = Multiply(x=w475, y=1.0) -> (x*y=w476:dbl)
      }
      frame "grande home" {
        w496 = FALSE
        # "Planta"
        n147 = Absolute Value(x=w495) -> (abs(x)=w500:dbl)
        n148 = local write "saturacion 2"(0.35) -> ()
        n149 = shared-variable ".\\RT Variables.lvlib\\Homing"(FALSE ("Homing")) -> ()  [unwired: 1 in, 1 out]
        n150 = Less?(x=w500, y=25.0) -> (x < y?=w491:bool)
        n151 = Select(t=T3."peque-sensor" ("Enum"), s=w491, f=T3."grande home" ("Enum")) -> (s? t:f=w503:T3)
        n152 = Absolute Value(x=w488) -> (abs(x)=w493:dbl)
        n153 = Multiply(x=w488, y=-1.0) -> (x*y=w489:dbl)
      }
      frame "peque-sensor" {
        w511 = TRUE
        # "sentido del pequeño esta en el grande"
        n154 = Select(t=T3."peque- home" ("Enum"), s=w510, f=T3."peque-sensor" ("Enum")) -> (s? t:f=w514:T3)
        n155 = Absolute Value(x=0.3 ("f")) -> (abs(x)=w508:dbl)
      }
      frame "peque- home" {
        n156 = Absolute Value(x=w519) -> (abs(x)=w524:dbl)
        n157 = Less?(x=w524, y=25.0) -> (x < y?=w522:bool)
        n158 = Select(t=T3."peque-reset" ("Enum"), s=w522, f=T3."peque- home" ("Enum")) -> (s? t:f=w527:T3)
        n159 = Absolute Value(x=-0.3 ("saturacion")) -> (abs(x)=w520:dbl)
      }
      frame "peque-reset" {
        w529 = TRUE
        n160 = Select(t=T3."normal" ("Enum"), s=w529, f=T3."peque-reset" ("Enum")) -> (s? t:f=w533:T3)
      }
    }
    n161 = Select(t=w193, s=w245, f=w158) -> (s? t:f=w246:dbl)
    n162 = Less Than 0?(x=w246) -> (x < 0?=w290:bool)
    n163 = Greater Or Equal To 0?(x=w246) -> (x >= 0?=w289:bool)
    n164 = xnode "Digital output (1 sample) 3"("A/DIO2 (Pin 15)"=w290) -> ()  [unwired: 1 in, 1 out]
    n165 = xnode "Digital output (1 sample) 4"("A/DIO3 (Pin 17)"=w289) -> ()  [unwired: 1 in, 1 out]
    n166 = Bundle(w188, "saturacion"=w190, w211, "seconds since 1Jan1904"=w344, w187, "saturacion 2"=w191, w159) -> (w213:T27)  [unwired: 1 in]
    n167 = local write "grandeoffset"(w197) -> ()
    n168 = local write "Reset Counter"(w307) -> ()
    n169 = local write "Reset Counter 2"(w305) -> ()
    n170 = local write "pequeoffset"(w196) -> ()
    n171 = Select(t=w192, s=w245, f=w169) -> (s? t:f=w279:dbl)
    n172 = xnode "Analog input (1 sample) 3"() -> ("stallBlanco (A/AI1 (Pin 5))"=w250:dbl, "stallRojo (A/AI0 (Pin 3))"=w252:dbl)  [unwired: 1 in, 1 out]
    "stallBlanco (A/AI1 (Pin 5))" <- w250
    "stallRojo (A/AI0 (Pin 3))" <- w252
    n173 = call <vilib>:"Set Duty Cycle.vi"("Duty Cycle"=w191, "PWM Ref In"=w314) -> ("error out"=w335:errorcluster, "PWM Ref Out"=w341:T5)  [unwired: 7 in]
    n174 = call <vilib>:"Set Duty Cycle.vi"("Duty Cycle"=w190, "PWM Ref In"=w337) -> ("error out"=w336:errorcluster, "PWM Ref Out"=w332:T5)  [unwired: 7 in]
    n175 = Multiply(x=0.987577800493881, y=w258) -> (x*y=w260:dbl)
    n176 = Multiply(x=0.012422199506119, y=w251) -> (x*y=w259:dbl)
    n177 = Multiply(x=0.987577800493881, y=w253) -> (x*y=w255:dbl)
    n178 = Multiply(x=0.012422199506119, y=w249) -> (x*y=w254:dbl)
    n179 = Add(x=w260, y=w259) -> (x+y=w248:dbl)
    n180 = Add(x=w255, y=w254) -> (x+y=w247:dbl)
    n181 = Merge Errors(w335, w336) -> (w334:errorcluster)
    n182 = shared-variable ".\\RT Variables.lvlib\\Stop RT Loops"() -> (w343:bool)  [unwired: 1 in, 1 out]
    n183 = Greater?(x=w248, y=0.2) -> (0:w317:bool)
    n184 = Greater?(x=w247, y=0.2) -> (0:w316:bool)
    n185 = shared-variable ".\\RT Variables.lvlib\\Data"(w213, error in=w334) -> (error out=w342:errorcluster)
    n186 = Or(x=w317, y=w316) -> (x .or. y?=w242:bool)
    n187 = Less Than 0?(x=w279) -> (x < 0?=w285:bool)
    n188 = Greater Or Equal To 0?(x=w279) -> (x >= 0?=w214:bool)
    n189 = Select(t=enum16{"No Stall", "Stall"}."Stall", s=w242, f=w238) -> (s? t:f=w241:enum16{"No Stall", "Stall"})
    n190 = Or(x=w342, y=w343) -> (x .or. y?=w331:bool)
    n191 = xnode "Digital output (1 sample)"("A/DIO0 (Pin 11)"=w285) -> ()  [unwired: 1 in, 1 out]
    n192 = xnode "Digital output (1 sample) 2"("A/DIO1 (Pin 13)"=w214) -> ()  [unwired: 1 in, 1 out]
    n193 = case shown="\"Stall\"" w241 {
      tunnel: [enum16{"No Stall", "Stall"}."No Stall" w390] -> w239
      tunnel: [FALSE ("stall") TRUE ("stall")] -> w237
      frame "No Stall", Default {
        # "aca quitaste lo de saturacion 0.7"
      }
      frame "Stall" {
        n194 = local write "saturacion"(0.0) -> ()
        n195 = feedback #2(0.0) -> (w397:dbl)
        n196 = Increment(x=w397) -> (x+1=w395:dbl)
        n197 = feedback-in #2(w395) -> ()
        n198 = Less?(x=1000.0, y=w395) -> (x < y?=w396:bool)
        n199 = Select(t=enum16{"No Stall", "Stall"}."No Stall", s=w396, f=enum16{"No Stall", "Stall"}."Stall") -> (s? t:f=w390:enum16{"No Stall", "Stall"})
      }
    }
    "stall" <- w237
    n200 = xnode "Button"() -> ("Value"=w243:bool)  [unwired: 1 in, 1 out]
    n201 = Or(x=w331, y=w243) -> (x .or. y?=w330:bool)
  }
  n202 = while {
    tunnel: [w830] -> w59
    shift-right: [w834] -> _
    shift-left: refnum<k21> refnum ("reader endpoint") -> [w832]
    shift-right: [w833] -> _
    shift-left: enum16{"Connect", "Receive"}."Connect" ("Message states") -> [w835]
    tunnel: w11 -> [w831]
    tunnel: w11 -> [w828]
    stop <- w829 stop-if-true
    # "Message loop"
    n203 = case shown="\"Receive\"" w835 {
      tunnel: [w842 w859] -> _
      tunnel: [w840 w871] -> w834
      tunnel: [w849 w868] -> w833
      tunnel: w832 -> [_ w867]
      tunnel: w831 -> [_ w870]
      tunnel: [FALSE ("Stop RT Loops") w869] -> w829
      tunnel: w828 -> [_ w864]
      tunnel: [_ w860] -> w827
      frame "Connect" {
        # "Attempts connection with the UI every 5 seconds, once successful, proceeds to Receive state."
        n204 = Bundle("", variant, variant) -> (w845:cluster{string, variant, variant})  [unwired: 1 in]
        n205 = Create Network Stream Reader Endpoint(5:5000 ("timeout in ms (-1)"), 7:4096 ("reader buffer size"), 9:w845, 11:"message reader" ("reader name")) -> (0:w844:errorcluster, 3:w839:refnum<k21>)  [unwired: 3 in]
        n206 = case shown="Error" w844 {
          selector: w844 -> [w854 _]
          tunnel: [enum16{"Connect", "Receive"}."Receive" ("Message states") enum16{"Connect", "Receive"}."Connect" ("Message states")] -> w849
          tunnel: [w853 errorcluster {"status"=FALSE, "code"=0, "source"=""} ("error IO")] -> w842
          tunnel: [w852 refnum<k21> refnum ("reader endpoint")] -> w840
          tunnel: w839 -> [w852 _]
          frame No Error {
            n207 = shared-variable ".\\RT Variables.lvlib\\2setpoint"(w852, error in=w854) -> (error out=w853:errorcluster)
          }
          frame Error {
          }
        }
      }
      frame "Receive" {
        # "Receives messages from the UI."
        n208 = shared-variable-read(w867, w870) -> (w866:refnum<k21>, w872:errorcluster, w863:cluster{string, variant, variant})  [unwired: 1 in, 1 out]
        n209 = Unbundle(w863) -> (w874:string, w873:variant, w865:variant)
        n210 = case shown="\"Homing\"" w874 {
          tunnel: w873 -> [_ w895 w910 w916 w934]
          tunnel: w872 -> [w879 w897 w899 w915 w928]
          tunnel: [w878 w892 w906 w917 _] -> w859
          tunnel: [refnum<k21> refnum ("reader endpoint") refnum<k21> refnum ("reader endpoint") w905 w923 w932] -> w871
          tunnel: w866 -> [w877 w891 w905 w923 w932]
          tunnel: [w875 w894 FALSE ("Stop RT Loops") FALSE ("Stop RT Loops") FALSE ("Stop RT Loops")] -> w869
          tunnel: [enum16{"Connect", "Receive"}."Connect" ("Message states") enum16{"Connect", "Receive"}."Receive" ("Message states") enum16{"Connect", "Receive"}."Receive" ("Message states") enum16{"Connect", "Receive"}."Receive" ("Message states") enum16{"Connect", "Receive"}."Receive" ("Message states")] -> w868
          tunnel: w865 -> [_ w887 w898 w919 w927]
          tunnel: w864 -> [_ w886 _ _ _]
          tunnel: [w875 _ _ _ w925] -> w862
          tunnel: [_ _ _ _ w924] -> w861
          frame "Disconnect UI", Default {
            w875 = FALSE ("Stop RT Loops")
            n211 = Destroy Stream Endpoint(8:w879, 11:w877) -> (0:w878:errorcluster)
          }
          frame "Stop" {
            n212 = Variant To Data(error in=w897, type=TRUE ("Stop RT Loops"), Variant=w895) -> (data=w894:bool, error out=w896:errorcluster)
            n213 = Variant To Data(error in=w886, type=TRUE ("Stop RT Loops"), Variant=w887) -> (data=w884:bool, error out=w888:errorcluster)
            n214 = shared-variable ".\\RT Variables.lvlib\\Stop RT Loops"(w894, error in=w896) -> (error out=w882:errorcluster)
            n215 = shared-variable ".\\RT Variables.lvlib\\Stop RT Loops"(w884, error in=w888) -> (error out=w883:errorcluster)
            n216 = Merge Errors(w882, w883) -> (w881:errorcluster)
            n217 = Destroy Stream Endpoint(8:w881, 11:w891) -> (0:w892:errorcluster)
          }
          frame "Update setpoint" {
            n218 = Variant To Data(error in=w899, type=0.0, Variant=w910) -> (data=w908:dbl, error out=w907:errorcluster)
            n219 = Variant To Data(error in=w899, type=0.0, Variant=w898) -> (data=w901:dbl, error out=w900:errorcluster)
            n220 = shared-variable ".\\RT Variables.lvlib\\Setpoint2"(w901, error in=w900) -> ()  [unwired: 1 out]
            n221 = shared-variable ".\\RT Variables.lvlib\\Setpoint"(w908, error in=w907) -> (error out=w906:errorcluster)
          }
          frame "Vector Setpoints" {
            n222 = Variant To Data(error in=w915, type=0.0, Variant=w919) -> (data=w918:dbl)  [unwired: 1 out]
            n223 = Variant To Data(error in=w915, type=dbl[][][] [], Variant=w916) -> (data=w913:dbl[][][])  [unwired: 1 out]
            "vectores" <- w913
            n224 = Index Array(array=w913) -> (element #1=w912:dbl[][], element #2=w911:dbl[][])  [unwired: 6 in]
            "subarray" <- w912
            "subarray 2" <- w911
            n225 = shared-variable "myRIO-1900\\Untitled Library 6.lvlib\\subarray"(w912) -> ()  [unwired: 1 in, 1 out]
            n226 = shared-variable "myRIO-1900\\Untitled Library 7.lvlib\\subarray 2"(w911) -> ()  [unwired: 1 in, 1 out]
            n227 = shared-variable ".\\RT Variables.lvlib\\Tiempo"(w918) -> (error out=w917:errorcluster)  [unwired: 1 in]
          }
          frame "Homing" {
            n228 = Variant To Data(error in=w928, type=0.0, Variant=w927) -> (data=→"data":dbl)  [unwired: 1 out]
            n229 = Variant To Data(error in=w928, type=TRUE, Variant=w934) -> (data=w925:bool, error out=w924:errorcluster)
          }
        }
        n230 = shared-variable ".\\RT Variables.lvlib\\Homing"(w862, error in=w861) -> (error out=w860:errorcluster)
      }
    }
    n231 = case shown="No Error" w827 {
      selector: w827 -> [w836 w837]
      tunnel: [w836 w837] -> w830
      frame No Error {
        # "No action required."
      }
      frame Error {
        # "Stops RT in case of error."
        n232 = shared-variable ".\\RT Variables.lvlib\\Stop RT Loops"(TRUE ("Stop RT Loops")) -> ()  [unwired: 1 in, 1 out]
      }
    }
  }
  n233 = Destroy Stream Endpoint(8:w63, 11:w62) -> (0:w60:errorcluster)
  n234 = node-c288(w66) -> ()  [unwired: 1 out]
  n235 = case shown="Error" w55 {
    selector: w55 -> [w935 w936]
    tunnel: [w935 w936] -> w17
    frame No Error {
      # "No action required."
    }
    frame Error {
      # "Destroys Message network stream to stop Message loop, in case of error."
      n236 = shared-variable ".\\RT Variables.lvlib\\2setpoint"() -> (w937:refnum<k21>)  [unwired: 1 in, 1 out]
      n237 = Destroy Stream Endpoint(11:w937) -> ()  [unwired: 1 in, 1 out]
    }
  }
  n238 = call <vilib>:"Stop.vi"("error in (no error)"=w17, "Encoder Ref In"=w47) -> ("error out"=w48:errorcluster, "Encoder Ref Out"=w49:T12)  [unwired: 8 in]
  n239 = call <vilib>:"Stop.vi"("error in (no error)"=w17, "Encoder Ref In"=w16) -> ("error out"=w19:errorcluster, "Encoder Ref Out"=w20:T12)  [unwired: 8 in]
  n240 = call <vilib>:"Close.vi"("error in (no error)"=w48, "Encoder Ref In"=w49) -> ("error out"=w42:errorcluster)  [unwired: 9 in]
  n241 = call <vilib>:"Close.vi"("error in (no error)"=w19, "Encoder Ref In"=w20) -> ("error out"=w18:errorcluster)  [unwired: 9 in]
  n242 = call <vilib>:"Close.vi"("error in (no error)"=w42, "PWM Ref In"=w39) -> ("error out"=w41:errorcluster)  [unwired: 9 in]
  n243 = call <vilib>:"Close.vi"("error in (no error)"=w18, "PWM Ref In"=w15) -> ("error out"=w14:errorcluster)  [unwired: 9 in]
  n244 = Merge Errors(w60, w59, w41, w14) -> (w58:errorcluster)
  n245 = shared-variable "myRIO-1900\\Network Shared Variables.lvlib\\error IO"(w58) -> ()  [unwired: 1 in, 1 out]
